vi "tx_init.vi"(8 "error in (no error)":errorcluster, 9 "Queues in":T4, 10 "HW parameters In":T3={"Device IP Address"="192.168.11.3", "Active Antenna"="TX1", "Carrier Frequency (Hz)"=915000000.0, "Gain (dB)"=10.0, "Generation Mode"=enum."continuous"} {"Gain (dB)" format="%.2f"; "Carrier Frequency (Hz)" format="%.2p"}, 11 "Modulation Parameters In":T2 {"TX Parameters"."TX Sample Rate" items=["4M"]}) -> (0 "error out":errorcluster, 1 "Queues out":T4, 2 "HW parameters out":T3={"Device IP Address"="192.168.11.3", "Active Antenna"="RF1", "Carrier Frequency (Hz)"=2400000000.0, "Gain (dB)"=10.0, "Generation Mode"=enum."single shot"} {"Gain (dB)" format="%.2f"; "Carrier Frequency (Hz)" format="%.2p"}, 3 "Modulation Parameters Out":T2 {"TX Parameters"."TX Sample Rate" items=["4M"]}, 4 "coerced gain (dB)":dbl format="%#_6f", 6 "coerced carrier frequency (Hz)":dbl=100000.0 format="%#_6p")   [LabVIEW 2012, in "gds_hw_config.lvlib"]
uses:
  EE 497/LABS/SDR/control_type_defs.llb/tx_hw params.ctl
  EE 497/LABS/SDR/control_type_defs.llb/Queues.ctl
  gds_hw_config.lvlib
panel:
  in  "Configurations Out":T1(tab)
  in  "Configuration In":T1(tab)
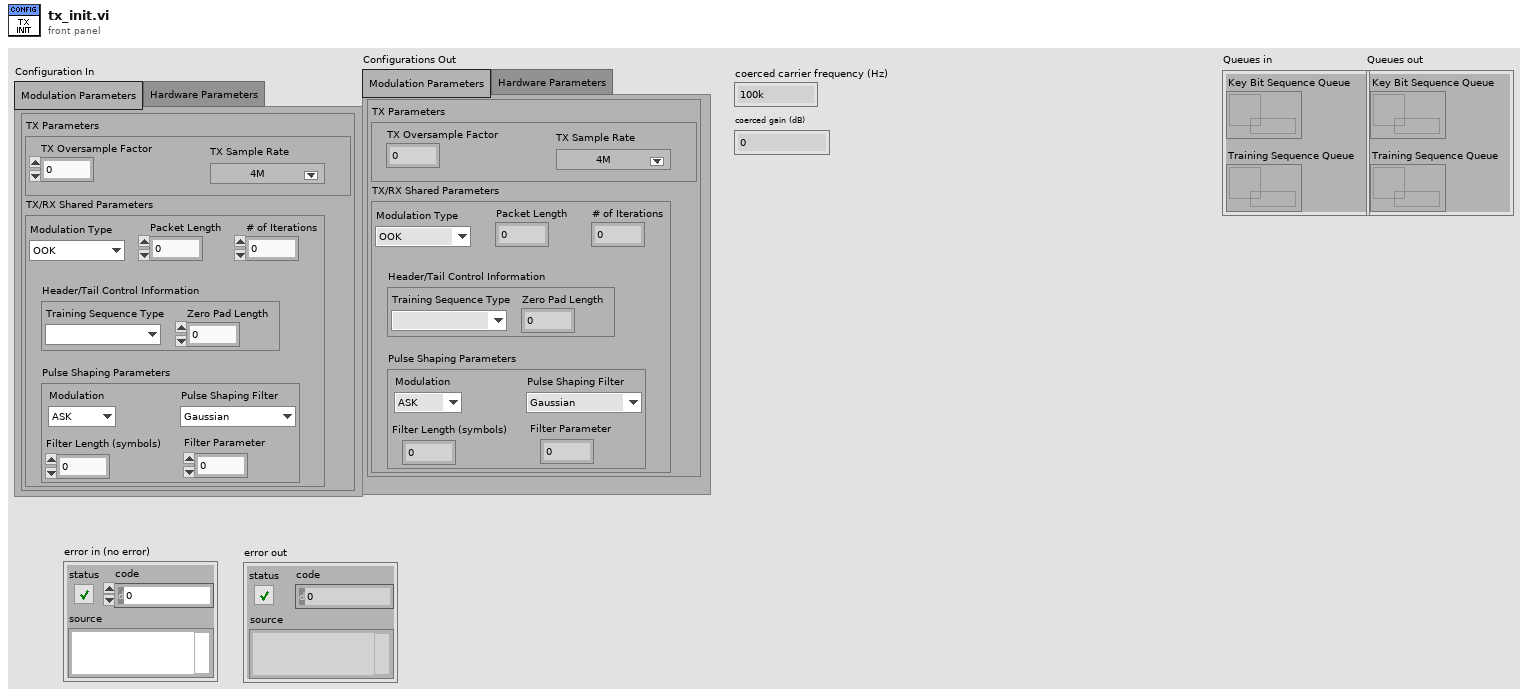
[diagram p1: front panel]
types:
  T1 = enum32{"Modulation Parameters", "Hardware Parameters"}
  T2 = cluster{"TX Parameters":cluster{"TX Oversample Factor":dbl, "TX Sample Rate":dbl}, "TX/RX Shared Parameters":cluster{"Modulation Type":enum16{"OOK", "FSK"}, "Packet Length":dbl, "# of Iterations":dbl, "Pulse Shaping Parameters":cluster{"Modulation":enum16{"ASK", "FSK", "PSK", "QAM", "MSK", "PAM"}, "Pulse Shaping Filter":enum16{"Gaussian"}, "Filter Length (symbols)":dbl, "Filter Parameter":dbl}, "Header/Tail Control Information":cluster{"Training Sequence Type":enum16{""}, "Zero Pad Length":dbl}}}
  T3 = typedef "tx_hw params.ctl" = cluster{"Device IP Address":refnum<k15>, "Active Antenna":string, "Carrier Frequency (Hz)":dbl, "Gain (dB)":dbl, "Generation Mode":enum16{"single shot", "simulate", "continuous"}}
  T4 = typedef "Queues.ctl" = cluster{"Key Bit Sequence Queue":refnum<queue>, "Training Sequence Queue":refnum<queue>}
  T5 = cluster{"TX Oversample Factor":dbl, "TX Sample Rate":dbl}
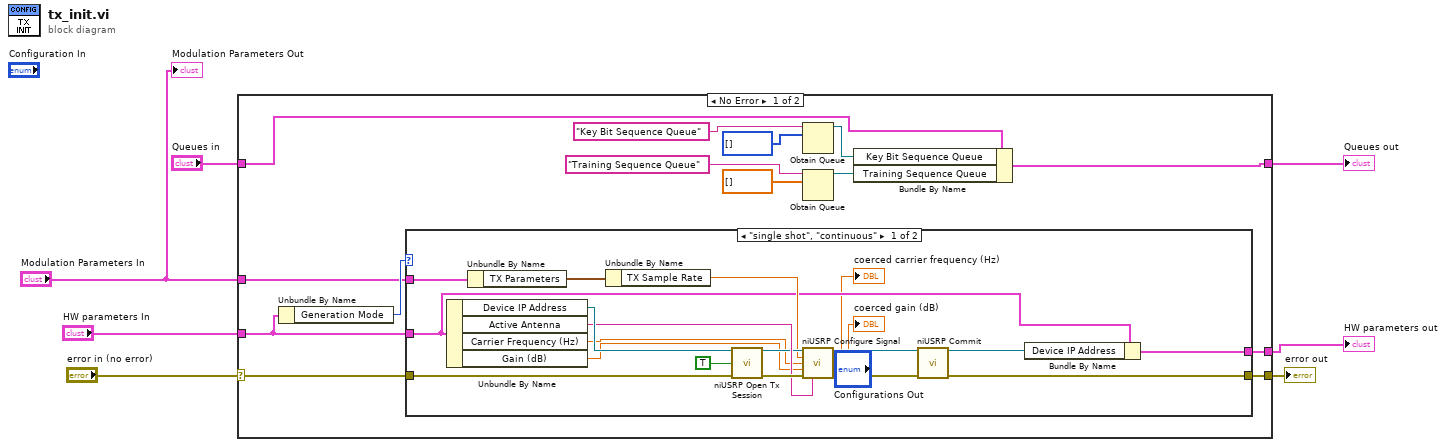
[diagram p0: block diagram]
diagram:
  n1 = case shown="No Error" "error in (no error)" {
    selector: "error in (no error)" -> [w18 w45]
    tunnel: [w17 w45] -> w6
    tunnel: [w20 w44] -> w5
    tunnel: "HW parameters In" -> [w19 w44]
    tunnel: "Modulation Parameters In" -> [w16 _]
    tunnel: "Queues in" -> [w9 w43]
    tunnel: [w8 w43] -> w2
    frame No Error {
      n2 = Unbundle By Name(w19) -> ("Generation Mode"=w21:enum16{"single shot", "simulate", "continuous"})
      n3 = case shown="\"single shot\", \"continuous\"" w21 {
        tunnel: [w24 w42] -> w20
        tunnel: w19 -> [w25 w42]
        tunnel: w18 -> [w40 w41]
        tunnel: [w27 w41] -> w17
        tunnel: w16 -> [w39 _]
        frame "single shot", "continuous" {
          n4 = Unbundle By Name(w25) -> ("Device IP Address"=w37:refnum<k15>, "Active Antenna"=w34:string, "Carrier Frequency (Hz)"=w32:dbl, "Gain (dB)"=w31:dbl)
          n5 = Unbundle By Name(w39) -> ("TX Parameters"=w38:T5)
          n6 = Unbundle By Name(w38) -> ("TX Sample Rate"=w30:dbl)
          n7 = call <instrlib>:"niUSRP Open Tx Session.vi"("device names"=w37, "reset"=TRUE, "error in (no error)"=w40) -> ("session handle out"=w33:refnum<k15>, "error out"=w35:errorcluster)  [unwired: 11 in]
          n8 = call <instrlib>:"niUSRP Configure Signal.vi"("session handle"=w33, "IQ rate"=w30, "carrier frequency"=w32, "gain"=w31, "error in (no error)"=w35, "active antenna"=w34) -> ("session handle out"=w29:refnum<k15>, "coerced carrier frequency"=→"coerced carrier frequency (Hz)":dbl, "coerced gain"=→"coerced gain (dB)":dbl, "error out"=w28:errorcluster)  [unwired: 5 in, 1 out]
          n9 = call <instrlib>:"niUSRP Commit.vi"("session handle"=w29, "error in (no error)"=w28) -> ("session handle out"=w26:refnum<k15>, "error out"=w27:errorcluster)  [unwired: 12 in]
          n10 = Bundle By Name(cluster=w25, "Device IP Address"=w26) -> (w24:T3)
        }
        frame "simulate", Default {
        }
      }
      n11 = Obtain Queue(name (unnamed)="Key Bit Sequence Queue", element data type=u8[] []) -> (queue out=w11:refnum<queue>)  [unwired: 3 in, 2 out]
      n12 = Obtain Queue(name (unnamed)="Training Sequence Queue", element data type=cdb[] []) -> (queue out=w10:refnum<queue>)  [unwired: 3 in, 2 out]
      n13 = Bundle By Name(cluster=w9, "Key Bit Sequence Queue"=w11, "Training Sequence Queue"=w10) -> (w8:T4)
    }
    frame Error {
    }
  }
  "error out" <- w6
  "HW parameters out" <- w5
  "Queues out" <- w2
  "Modulation Parameters Out" <- "Modulation Parameters In"
